vi "forleercadatanto.vi"() -> ()   [LabVIEW 2018]
uses:
  <vilib>/Utility/file.llb/Read Delimited Spreadsheet (DBL).vi
panel:
  in  "tiempo":dbl
  out "element":dbl
  out "element 2":dbl
  in  "Stop UI":bool
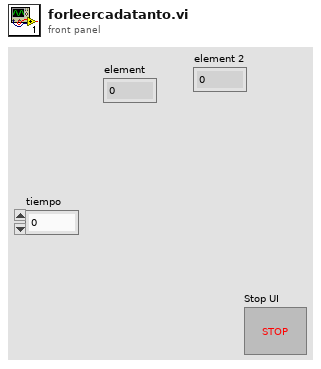
[diagram p1: front panel]
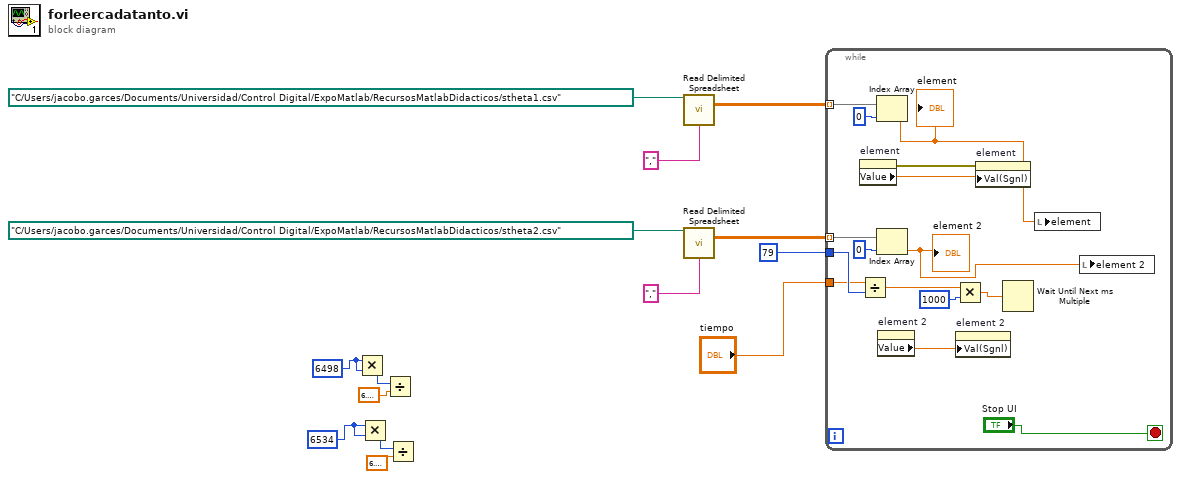
[diagram p0: block diagram]
diagram:
  w1 = 6534
  w2 = 6498
  n1 = Multiply(x=w2, y=w2) -> (x*y=w5:i32)
  n2 = Multiply(x=w1, y=w1) -> (x*y=w6:i32)
  n3 = Divide(x=w5, y=6.283185307179586) -> ()  [unwired: 1 out]
  n4 = Divide(x=w6, y=6.283185307179586) -> ()  [unwired: 1 out]
  n5 = call-poly <vilib>:"Read Delimited Spreadsheet.vi"("file path (dialog if empty)"=path "C:/Users/jacobo.garces/Documents/Universidad/Control Digital/ExpoMatlab/RecursosMatlabDidacticos/stheta1.csv", "delimiter (\\t)"="," ("delimiter (\\t)")) -> ("all rows"=w12:dbl[][])  [unwired: 8 in, 5 out]
  n6 = call-poly <vilib>:"Read Delimited Spreadsheet.vi"("file path (dialog if empty)"=path "C:/Users/jacobo.garces/Documents/Universidad/Control Digital/ExpoMatlab/RecursosMatlabDidacticos/stheta2.csv", "delimiter (\\t)"="," ("delimiter (\\t)")) -> ("all rows"=w13:dbl[][])  [unwired: 8 in, 5 out]
  n7 = while {
    tunnel: 79 -> [w27]
    tunnel: w12 -> [w26] mode=indexing
    tunnel: "tiempo" -> [w24]
    tunnel: w13 -> [w22] mode=indexing
    stop <- "Stop UI" stop-if-true
    n8 = property on="element" class="DigNum (strict)"() -> (error out=w20:errorcluster, "Value"=w21:dbl)  [unwired: 2 in, 1 out]
    n9 = Divide(x=w24, y=w27) -> (x/y=w29:dbl)
    n10 = Index Array(array=w26, index=0) -> (element=w19:dbl)
    "element" <- w19
    n11 = Index Array(array=w22, index=0) -> (element=w16:dbl)
    "element 2" <- w16
    n12 = property on="element 2" class="DigNum (strict)"() -> ("Value"=w18:dbl)  [unwired: 2 in, 2 out]
    n13 = Multiply(x=w29, y=1000) -> (x*y=w17:dbl)
    n14 = property on="element 2" class="DigNum (strict)"("Val(Sgnl)"=w18) -> ()  [unwired: 2 in, 2 out]
    n15 = property on="element" class="DigNum (strict)"(error in=w20, "Val(Sgnl)"=w21) -> ()  [unwired: 1 in, 2 out]
    n16 = Wait Until Next ms Multiple(millisecond multiple=w17) -> ()  [unwired: 1 out]
    n17 = local write "element"(w19) -> ()
    n18 = local write "element 2"(w16) -> ()
  }
